vi "DP I-O (Bias).vi"(11 "Expt State (in)":T6) -> (3 "State":T6)   [LabVIEW 2020]
uses:
  CFTS Main Panel SubVIs/CFTS-Data Type Enum.ctl
  Utility VIs/Type Defs/Left-Right ring.ctl
  CFTS Main Panel SubVIs/CFTS-Experiment State.ctl
  Typedefs/DP-StimGen.ctl
  Typedefs/DP-Rejection Settings.ctl
  Typedefs/DP-Stim Params (F1L1).ctl
panel:
  in  "Tab Control":enum32{"Probe tones", "Bias tone"}(tab)
  in  "DP Params":T1={"Start (dB)"=20.0, "Stop (dB)"=70.0, "Step (dB)"=10.0, "Ear"=enum."Right", "f2 (kHz)"="5.6;8.0;11.3;16;22.6;32;", "f1"=1.2, "f1 mode"=enum."re f2", "L1"=10.0, "L1 mode"=enum."re L2"}
  in  "Reject":T3 caption="Rejection"
  in  "StimGen":T4={"Sampling Rate (Hz)"=200000.0, "Npts"=10000, "Data Folder"=path "", "Acoustic System"="", "Recalibrate?"=FALSE, "AO Channels"=[], "Mic  gain (dB)"=0.0, "F1, F2 speakers"=[], "Override recal check"=FALSE}
  out "Freqs":cluster{"f1":dbl, "f2":dbl, "2f1-f2":dbl}={"f1"=9419.759114583332, "f2"=11291.50390625, "2f1-f2"=7548.014322916664} {"2f1-f2" format="%.3f"; "f1" format="%.3f"; "f2" format="%.3f"}
  out "Abort":bool
  in  "Recalibrate":bool
  in  "Probe Mic Gain (dB)":dbl
  in  "Save Waves?":bool=TRUE
  out "User":string
  out "Run #":u16=14
  out "ID #":u16=1
  in  "Avg specs":T5={"# Time avgs "=8, "# Spectrum avgs"=4}
  out "running":bool
  out "Path":path
  out "DP window":cluster{i32, "df (Hz)":dbl, dbl[]}(graph)={0, "df (Hz)"=0.02, []}
  out "I-O Plot":cluster{cluster{dbl, dbl}[]}[](graph)
  in  "Notes":string
  out "Full Spectrum":cluster{i32, "Freq Resolution":dbl, dbl[]}(graph)={0, "Freq Resolution"=20.345052083333332, []}
  in  "RETURN":bool
  in  "START":bool
  in  "STOP":bool
  # "Averaging"
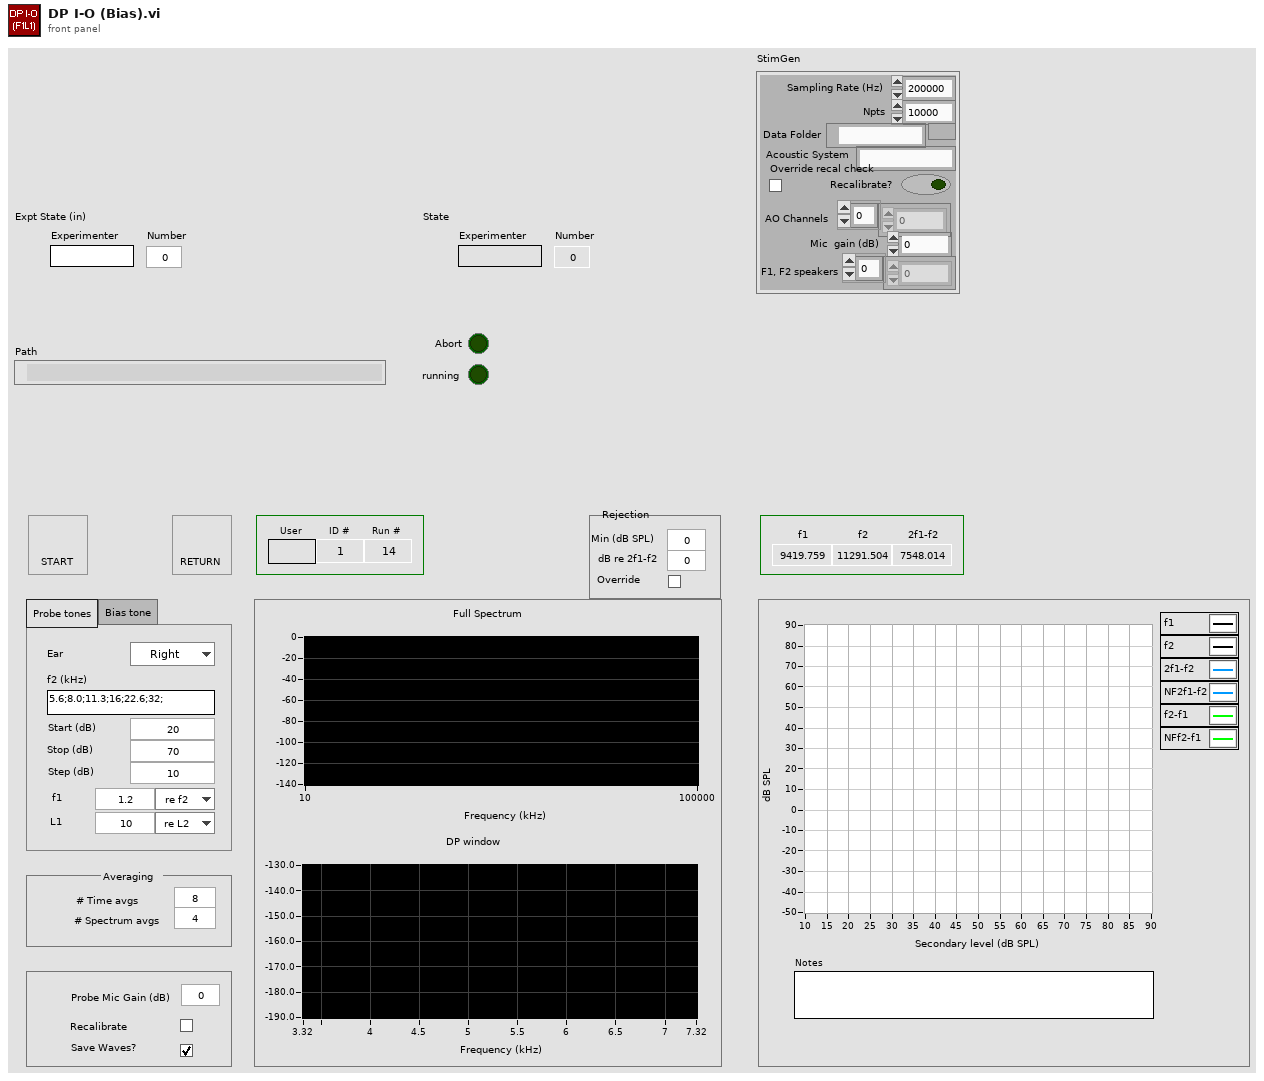
[diagram p1: front panel]
types:
  T1 = typedef "DP-Stim Params (F1L1).ctl" = cluster{"Start (dB)":dbl, "Stop (dB)":dbl, "Step (dB)":dbl, "Ear":T2, "f2 (kHz)":string, "f1":dbl, "f1 mode":enum16{"re f2", "kHz"}, "L1":dbl, "L1 mode":enum16{"re L2", "dB"}}
  T2 = typedef "Left-Right ring.ctl" = enum16{"Right", "Left"}
  T3 = typedef "DP-Rejection Settings.ctl" = cluster{"Override":bool, "dB re 2f1-f2":dbl, "Min (dB SPL)":dbl}
  T4 = typedef "DP-StimGen.ctl" = cluster{"Sampling Rate (Hz)":dbl, "Npts":i32, "Data Folder":path, "Acoustic System":string, "Recalibrate?":bool, "AO Channels":i32[], "Mic  gain (dB)":dbl, "F1, F2 speakers":i32[], "Override recal check":bool}
  T5 = cluster{"# Time avgs ":i32, "# Spectrum avgs":i32}
  T6 = typedef "CFTS-Experiment State.ctl" = cluster{"Experimenter":string, "Number":u32, "Right":string, "Left":string, "Data Folder":path, "State File":path, "Version Info":string, "End Exposure Time":dbl, "Exposure Duration":string, "Run #":cluster{"CAP":i16, "ABR":i16, "DP":i16, "VsEP":i16, "MeasSeq":i16, "SubSeq":i16, "SFOAE":i16}}
  T7 = typedef "CFTS-Data Type Enum.ctl" = enum16{"CAP", "ABR", "DP", "VsEP", "MeasSeq", "SFOAE"}
  T8 = typedef "DP-Freqs.ctl" = cluster{"f1":dbl, "f2":dbl, "2f1-f2":dbl}
  T9 = typedef "DP-DataAcq.ctl" = cluster{"#spectra avgs":i32[], "#time avgs":i32[], "dt (ms)":dbl, "df (kHz)":dbl, "Npts":i32, "Save waves?":bool, "Data File":path, "AI Channels":u16[], "Sampling rate (Hz)":dbl, "Probe Tube Sensitivity":cluster{"Frequency":dbl[], "Mag":dbl[]}, "Mic gain (dB)":dbl, "ptIndex":i32}
  T10 = typedef "CFTS-Options.ctl" = cluster{"DP Artifact Rejection":bool, "Monitor vital signs ":bool, "Extension":string}
  T11 = cluster{"Shift":bool, "Ctrl":bool, "Alt":bool, "Cmd":bool, "Opt":bool}
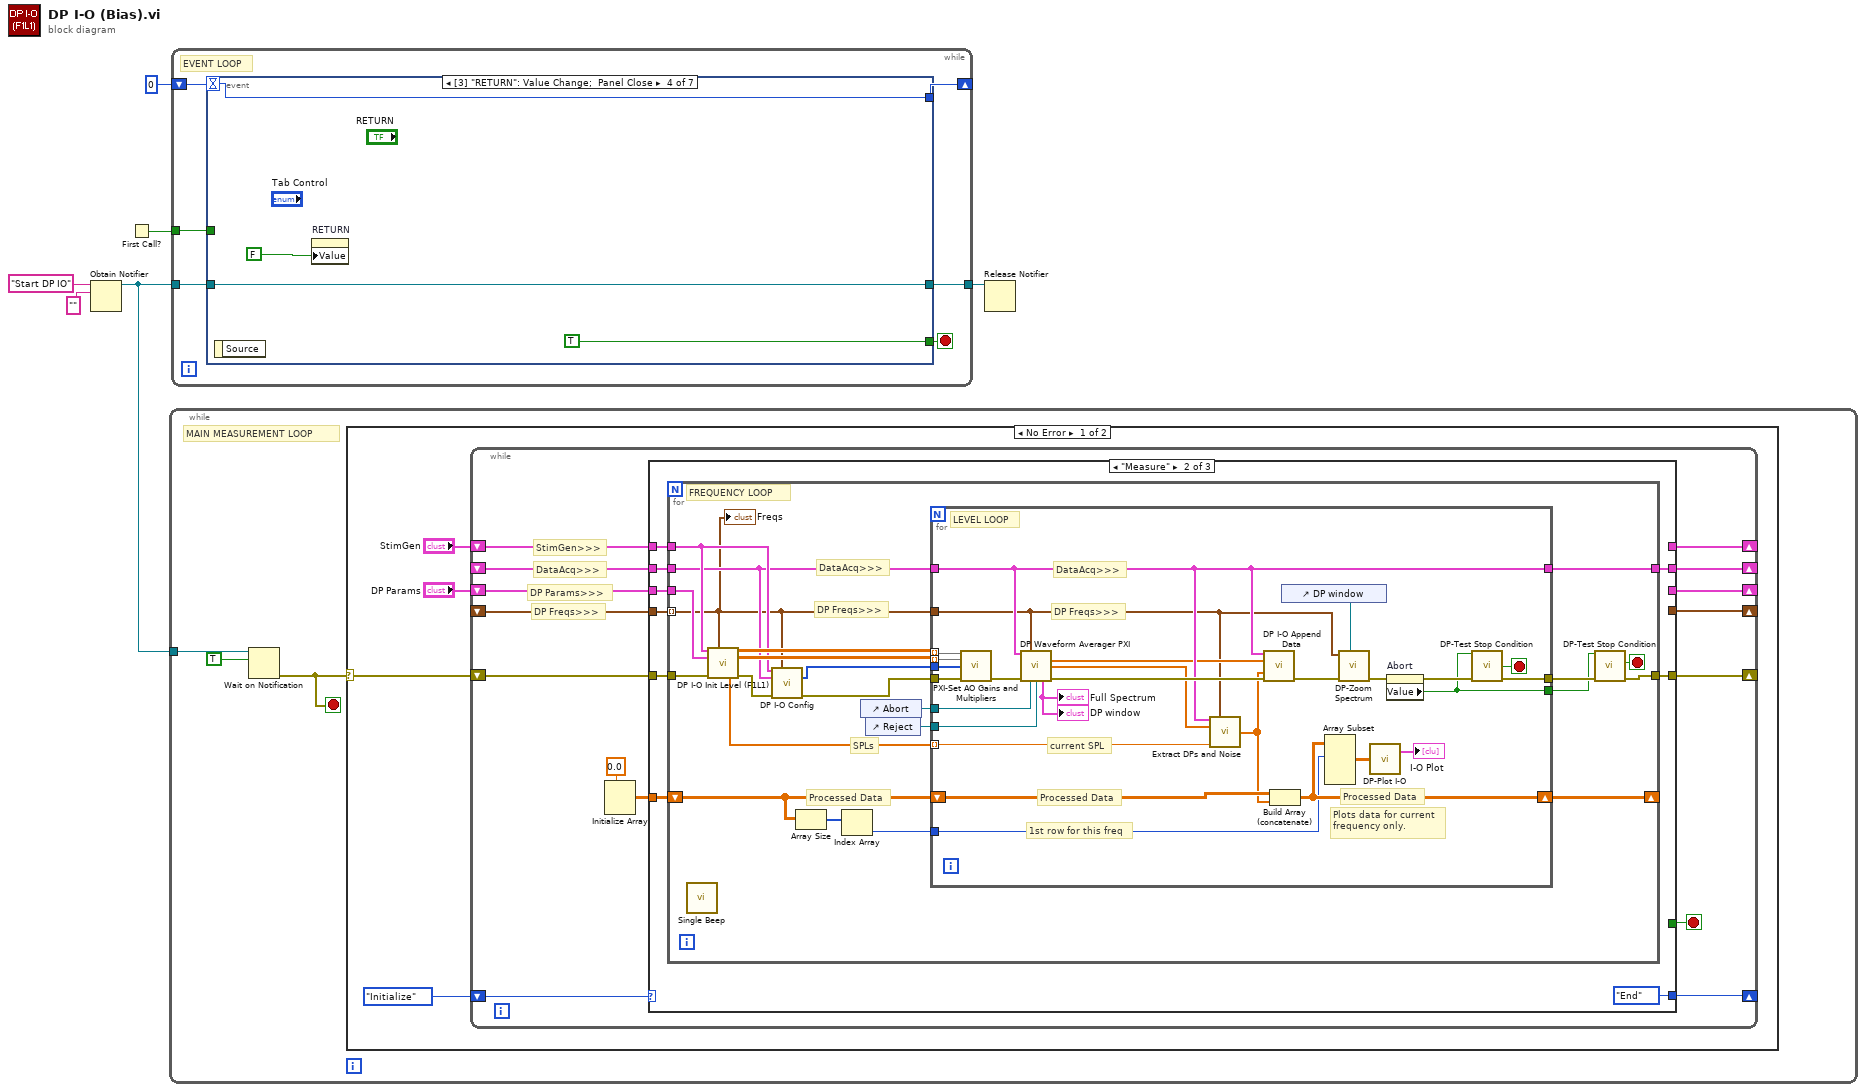
[diagram p0: block diagram]
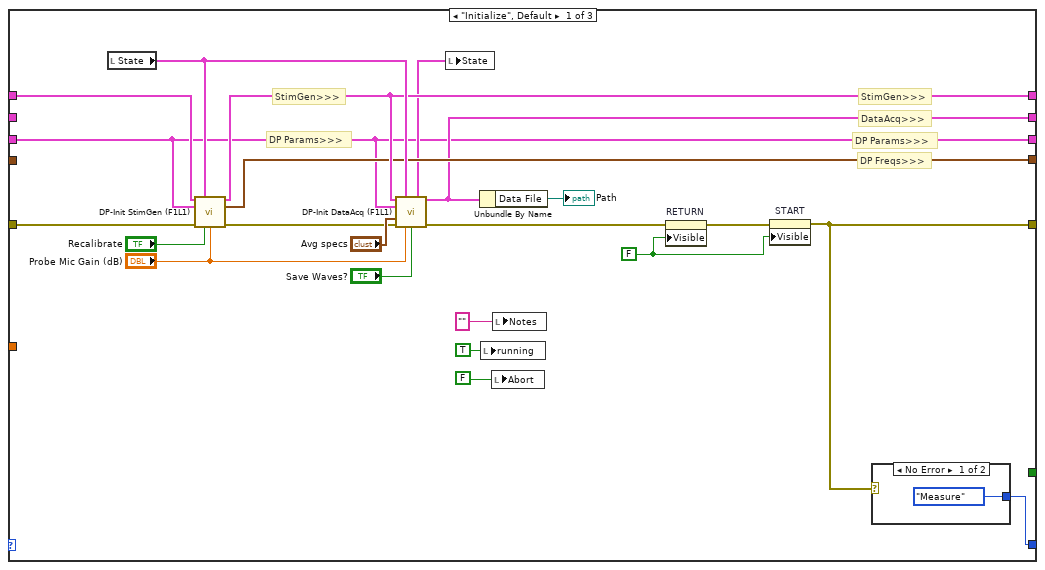
[diagram p2: hidden frame]
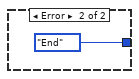
[diagram p3: hidden frame]
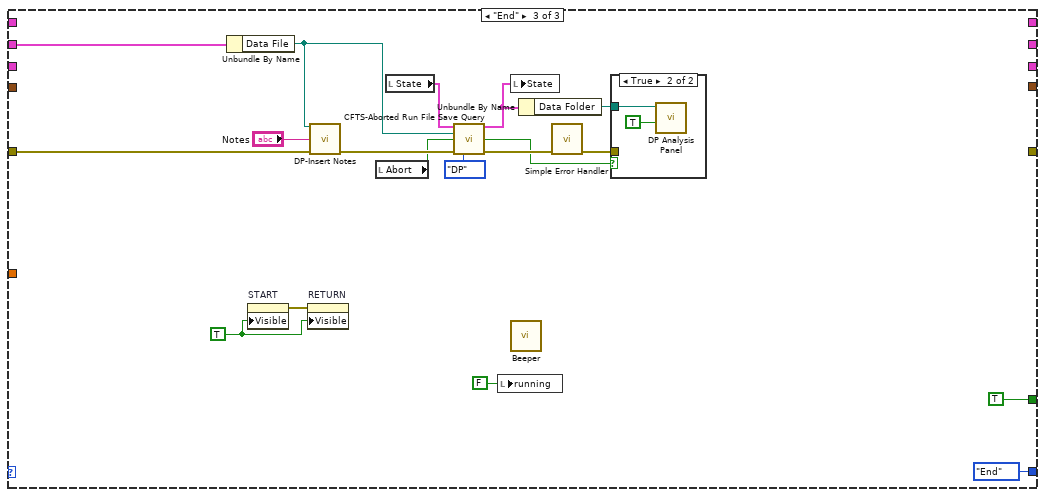
[diagram p4: hidden frame]
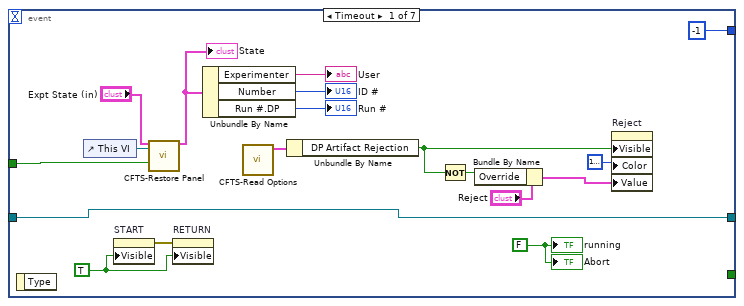
[diagram p7: hidden frame]
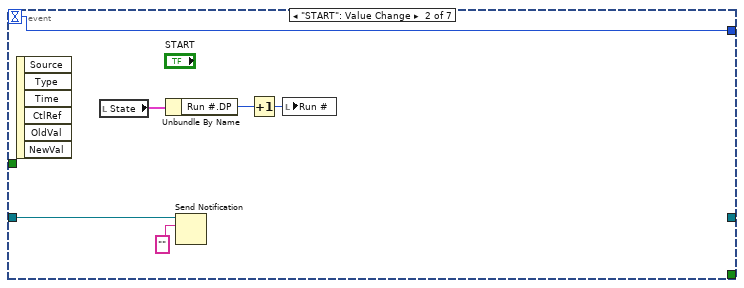
[diagram p8: hidden frame]
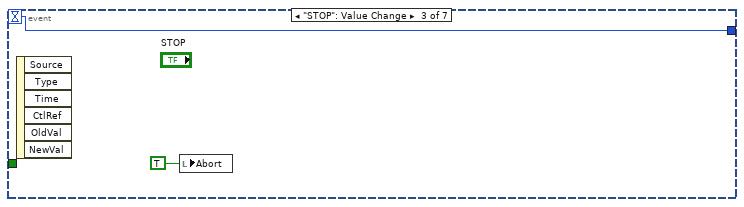
[diagram p9: hidden frame]
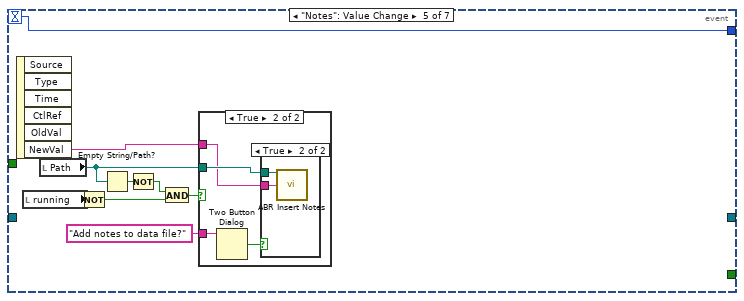
[diagram p10: hidden frame]
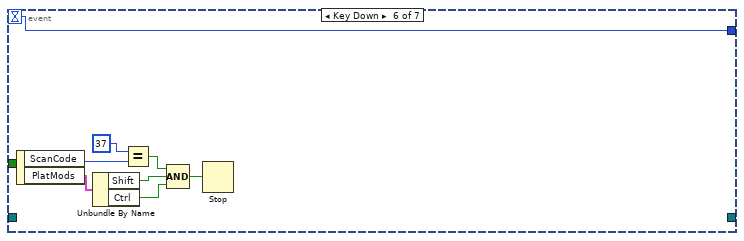
[diagram p13: hidden frame]
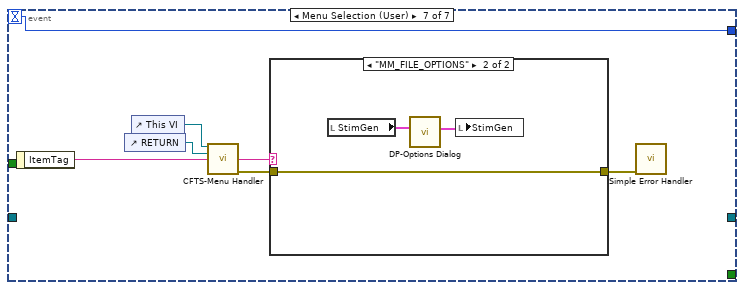
[diagram p14: hidden frame]
diagram:
  n1 = Obtain Notifier(name (unnamed)="Start DP IO", notification data type="") -> (notifier out=w6:refnum<notifier>)  [unwired: 2 in, 2 out]
  n2 = First Call?() -> (First Call?: T/F=w1:bool)
  n3 = while {
    tunnel: w6 -> [w8]
    stop <- w7 stop-if-true
    # "MAIN MEASUREMENT LOOP"
    n4 = Wait on Notification(notifier=w8, ignore previous (F)=TRUE) -> (error out=w7:errorcluster)  [unwired: 2 in, 3 out]
    n5 = case shown="No Error" w7 {
      selector: w7 -> [w10 _]
      frame No Error {
        n6 = while {
          shift-right: [w27] -> _
          shift-left: w10 -> [w28]
          shift-right: [w18] -> _
          shift-left: enum16{"Initialize", "Measure", "End"}."Initialize" -> [w26]
          shift-right: [w22] -> _
          shift-left: "StimGen" -> [w24]
          shift-right: [w21] -> _
          shift-left: _ -> [w23]
          shift-right: [w19] -> _
          shift-left: "DP Params" -> [w20]
          shift-right: [w17] -> _
          shift-left: _ -> [w16]
          stop <- w25 stop-if-true
          # "DP Freqs>>>"
          # "DP Params>>>"
          # "DataAcq>>>"
          # "StimGen>>>"
          n7 = Initialize Array(0.0) -> (w14:dbl[][])  [unwired: 2 in]
          n8 = case shown="\"Measure\"" w26 {
            tunnel: w28 -> [w41 w61 w120]
            tunnel: [w31 w60 _] -> w27
            tunnel: [_ _ TRUE] -> w25
            tunnel: w24 -> [w43 w57 _]
            tunnel: w23 -> [_ w55 w121]
            tunnel: [w42 _ _] -> w22
            tunnel: [w33 w53 _] -> w21
            tunnel: w20 -> [w29 w56 _]
            tunnel: [w29 _ _] -> w19
            tunnel: [w30 enum16{"Initialize", "Measure", "End"}."End" enum16{"Initialize", "Measure", "End"}."End"] -> w18
            tunnel: [w36 _ _] -> w17
            tunnel: w16 -> [_ w58 _]
            tunnel: w14 -> [_ w59 _]
            frame "Initialize", Default {
              w47 = FALSE
              # "DP Freqs>>>"
              # "DP Params>>>"
              # "StimGen>>>"
              # "DP Params>>>"
              # "DataAcq>>>"
              # "StimGen>>>"
              n9 = local read "State"() -> (w44:T6)
              n10 = call "DP-Init StimGen (F1L1).vi"("StimGen"=w43, "Expt State"=w44, "DP stimulus params"=w29, "error in (no error)"=w41, "Recalibrate?"="Recalibrate", "Mic  gain (dB)"="Probe Mic Gain (dB)") -> ("StimGen (out)"=w42:T4, "DP Freqs"=w36:T8[], "error out"=w40:errorcluster)  [unwired: 7 in]
              n11 = call "DP-Init DataAcq (F1L1).vi"("StimGen"=w42, "Expt State"=w44, "DP stimulus params"=w29, "Avg specs"="Avg specs", "error in (no error)"=w40, "Mic gain (dB)"="Probe Mic Gain (dB)", "Save waves?"="Save Waves?") -> ("Expt State out"=w34:T6, "DataAcq"=w33:T9, "error out"=w38:errorcluster)  [unwired: 6 in]
              n12 = local write "State"(w34) -> ()
              n13 = Unbundle By Name(w33) -> ("Data File"=→"Path":path)
              n14 = local write "running"(TRUE ("running")) -> ()
              n15 = local write "Abort"(FALSE ("Stopping")) -> ()
              n16 = local write "Notes"("" ("Notes")) -> ()
              n17 = property on="RETURN" class="Bool (strict)"(error in=w38, "Visible"=w47) -> (error out=w37:errorcluster)  [unwired: 1 in, 1 out]
              n18 = property on="START" class="Bool"(error in=w37, "Visible"=w47) -> (error out=w31:errorcluster)  [unwired: 1 in, 1 out]
              n19 = case shown="No Error" w31 {
                tunnel: [enum16{"Initialize", "Measure", "End"}."Measure" enum16{"Initialize", "Measure", "End"}."End"] -> w30
                frame No Error {
                }
                frame Error {
                }
              }
            }
            frame "Measure" {
              n20 = for {
                shift-right: [w74] -> _
                shift-left: w59 -> [w81]
                tunnel: w61 -> [w78]
                tunnel: [w65] -> w60
                tunnel: w58 -> [w69] mode=indexing
                tunnel: w57 -> [w71]
                tunnel: w56 -> [w73]
                tunnel: w55 -> [w70]
                tunnel: [w68] -> w53
                stop <- w72 stop-if-true
                # "DP Freqs>>>"
                # "DataAcq>>>"
                # "FREQUENCY LOOP"
                # "Processed Data"
                # "SPLs"
                n21 = call "Single Beep.vi"() -> ()  [unwired: 1 in]
                n22 = call "DP I-O Init Level (F1L1).vi"("StimGen"=w71, "DP Freqs"=w69, "DP stimulus params"=w73, "error in (no error)"=w78) -> ("Multipliers (2D)"=w83:dbl[][], "Gains (2D)"=w82:dbl[][], "Nominal f2 SPL"=w75:dbl[], "error out"=w77:errorcluster)  [unwired: 7 in, 1 out]
                n23 = call "DP I-O Config.vi"("StimGen"=w71, "DP Freqs"=w69, "DataAcq"=w70, "error in (no error)"=w77) -> ("AO Channels"=w67:i32[], "error out"=w76:errorcluster)  [unwired: 10 in]
                n24 = Array Size(array=w81) -> (size(s)=w80:i32[])
                n25 = Index Array(array=w80) -> (element=w79:i32)  [unwired: 1 in]
                n26 = control-ref of="Abort"() -> (w63:refnum<vi>)
                n27 = control-ref of="Reject"() -> (w62:refnum<vi>)
                n28 = for {
                  tunnel: w83 -> [w109] mode=indexing
                  tunnel: w82 -> [w108] mode=indexing
                  tunnel: w75 -> [w95] mode=indexing
                  shift-right: [w105] -> w74
                  shift-left: w81 -> [w107]
                  tunnel: w79 -> [w103]
                  tunnel: w76 -> [w110]
                  tunnel: [w90] -> w66
                  tunnel: w70 -> [w94]
                  tunnel: w69 -> [w86]
                  tunnel: [w94] -> w68
                  tunnel: w67 -> [w91]
                  tunnel: [w87] -> w64
                  tunnel: w63 -> [w85]
                  tunnel: w62 -> [w84]
                  stop <- w101 stop-if-true
                  # "DP Freqs>>>"
                  # "DataAcq>>>"
                  # "LEVEL LOOP"
                  # "current SPL"
                  # "Plots data for current\nfrequency only."
                  # "1st row for this freq"
                  # "Processed Data"
                  # "Processed Data"
                  n29 = call "PXI-Set AO Gains and Multipliers.vi"("Multipliers"=w109, "Gains"=w108, "AO Channels"=w91, "error in (no error)"=w110) -> ("error out"=w100:errorcluster)  [unwired: 11 in]
                  n30 = call "DP Waveform Averager PXI.vi"("DataAcq"=w94, "DP Freqs"=w86, "error in"=w100, "Abort"=w85, "Reject Ref"=w84) -> ("Ave Wave"=w93:dbl[], "Averaged Spectrum (Vrms)"=w97:dbl[], "waveform cluster"=→"Full Spectrum" →"DP window":cluster{i32, "dx":dbl, "Array":dbl[]}, "error out"=w99:errorcluster)  [unwired: 5 in, 2 out]
                  n31 = call "Extract DPs and Noise.vi"("DataAcq"=w94, "DP Freqs"=w86, "Spectrum in Vrms"=w97, "SPL"=w95) -> ("Output Array"=w96:dbl[])  [unwired: 11 in]
                  n32 = call "DP I-O Append Data.vi"("DataAcq"=w94, "Waveform"=w93, "Processed data"=w96, "error in (no error)"=w99) -> ("error out"=w102:errorcluster)  [unwired: 11 in]
                  n33 = Build Array (concatenate)(w107, w96) -> (w105:dbl[][])
                  n34 = control-ref of="DP window"() -> (w92:refnum<vi>)
                  n35 = Array Subset(array=w105, index (row)=w103) -> (w104:dbl[][])  [unwired: 3 in]
                  n36 = call "DP-Zoom Spectrum.vi"("DP window"=w92, "error in (no error)"=w102, "DP Freqs"=w86) -> ("error out"=w89:errorcluster)  [unwired: 8 in]
                  n37 = call "DP-Plot I-O.vi"("Input Array (4xn)"=w104) -> ("Current I-O Plot"=→"I-O Plot":cluster{cluster{dbl, dbl}[]}[])  [unwired: 1 out]
                  n38 = property on="Abort" class="Bool (strict)"(error in=w89) -> (error out=w88:errorcluster, "Value"=w87:bool)  [unwired: 1 in, 1 out]
                  n39 = call "DP-Test Stop Condition.vi"("Abort?"=w87, "error in (no error)"=w88) -> ("Stop?"=w101:bool, "error out"=w90:errorcluster)  [unwired: 12 in]
                }
                n40 = call "DP-Test Stop Condition.vi"("Abort?"=w64, "error in (no error)"=w66) -> ("Stop?"=w72:bool, "error out"=w65:errorcluster)  [unwired: 12 in]
                "Freqs" <- w69
              }
            }
            frame "End" {
              w127 = TRUE
              n41 = Unbundle By Name(w121) -> ("Data File"=w117:path)
              n42 = property on="START" class="Bool"("Visible"=w127) -> (error out=w123:errorcluster)  [unwired: 2 in, 1 out]
              n43 = property on="RETURN" class="Bool (strict)"(error in=w123, "Visible"=w127) -> ()  [unwired: 1 in, 2 out]
              n44 = call "DP-Insert Notes.vi"("path"=w117, "Notes"="Notes", "error in (no error)"=w120) -> ("error out"=w122:errorcluster)  [unwired: 12 in]
              n45 = local read "Abort"() -> (w115:bool)
              n46 = local read "State"() -> (w118:T6)
              n47 = call "CFTS-Aborted Run File Save Query.vi"("Expt State"=w118, "Path"=w117, "Aborted"=w115, "error in (no error)"=w122, "Data Type"=CFTS-Data_Type_Enum."DP") -> ("Expt State out"=w114:T6, "File saved?"=w112:bool, "error out"=w119:errorcluster)  [unwired: 8 in]
              n48 = local write "running"(FALSE ("running")) -> ()
              n49 = local write "State"(w114) -> ()
              n50 = call "Beeper.vi"() -> ()  [unwired: 1 in]
              n51 = Unbundle By Name(w114) -> ("Data Folder"=w113:path)
              n52 = call <vilib>:"Simple Error Handler.vi"("error in (no error)"=w119) -> ("error out"=w111:errorcluster)  [unwired: 4 in, 4 out]
              n53 = case shown="True" w112 {
                tunnel: w113 -> [_ w130]
                tunnel: w111 -> [_ _]
                frame False {
                }
                frame True {
                  n54 = call "DP Analysis Panel.vi"("Autosave? (F)"=TRUE, "Data folder in"=w130) -> ()  [unwired: 10 in]
                }
              }
            }
          }
        }
      }
      frame Error {
      }
    }
  }
  n55 = while {
    tunnel: w6 -> [w136]
    shift-right: [w133] -> _
    shift-left: 0 -> [w134]
    tunnel: [w132] -> w2
    tunnel: w1 -> [w131]
    stop <- w135 stop-if-true
    # "EVENT LOOP"
    n56 = event shown="[3] \"RETURN\": Value Change;  Panel Close" {
      selector: _ -> [_ _ _ _ _ _ _]
      dyn-events: _ -> [_ _ _ _ _ _ _]
      timeout: w134 -> [_ w155 w162 w165 w167 w189 w196]
      tunnel: w136 -> [w147 w160 _ w164 _ _ _]
      tunnel: [_ _ _ TRUE _ _ _] -> w135
      tunnel: [-1 w155 w162 w165 w167 w189 w196] -> w133
      tunnel: [w147 _ _ w164 _ _ _] -> w132
      tunnel: w131 -> [w146 _ _ _ _ _ _]
      event Timeout {
        w150 = TRUE
        w149 = FALSE ("quitting")
        n57 = event-data() -> ()  [unwired: 1 in, 1 out]
        n58 = control-ref of="This VI"() -> (w145:refnum<vi>)
        n59 = property on="START" class="Bool"("Visible"=w150) -> (error out=w148:errorcluster)  [unwired: 2 in, 1 out]
        n60 = call "CFTS-Restore Panel.vi"("State (in)"="Expt State (in)", "VI refnum"=w145, "Restore?"=w146) -> ("State"=w143:T6)  [unwired: 11 in, 1 out]
        "State" <- w143
        n61 = property on="RETURN" class="Bool (strict)"(error in=w148, "Visible"=w150) -> ()  [unwired: 1 in, 2 out]
        n62 = Unbundle By Name(w143) -> ("Experimenter"=→"User":string, "Number"=→"ID #":u32, "Run #.DP"=→"Run #":i16)
        n63 = call "CFTS-Read Options.vi"() -> ("CFTS Options"=w142:T10)  [unwired: 10 in, 1 out]
        n64 = Unbundle By Name(w142) -> ("DP Artifact Rejection"=w138:bool)
        n65 = Not(x=w138) -> (.not. x?=w139:bool)
        n66 = Bundle By Name(cluster="Reject", "Override"=w139) -> (w137:T3)
        n67 = property on="Reject" class="Clust (strict)"("Visible"=w138, "Color"=u32 16777238, "Value"=w137) -> ()  [unwired: 2 in, 2 out]
        "running" <- w149
        "Abort" <- w149
      }
      event "START": Value Change {
        n68 = event-data() -> ()  [unwired: 1 in, 6 out]
        n69 = local read "State"() -> (w157:T6)
        n70 = Unbundle By Name(w157) -> ("Run #.DP"=w156:i16)
        n71 = Send Notification(notification="", notifier=w160) -> ()  [unwired: 1 in, 2 out]
        n72 = Increment(x=w156) -> (x+1=w158:i16)
        n73 = local write "Run #"(w158) -> ()
      }
      event "STOP": Value Change {
        n74 = event-data() -> ()  [unwired: 1 in, 6 out]
        n75 = local write "Abort"(TRUE ("Stopping")) -> ()
      }
      event "RETURN": Value Change; Panel Close {
        n76 = event-data() -> ()  [unwired: 1 in, 1 out]
        n77 = property on="RETURN" class="Bool (strict)"("Value"=FALSE) -> ()  [unwired: 2 in, 2 out]
      }
      event "Notes": Value Change {
        n78 = event-data() -> ("NewVal"=w170:string)  [unwired: 1 in, 5 out]
        n79 = local read "running"() -> (w168:bool)
        n80 = local read "Path"() -> (w169:path)
        n81 = Not(x=w168) -> (.not. x?=w172:bool)
        n82 = Empty String/Path?(string/path=w169) -> (empty?=w171:bool)
        n83 = Not(x=w171) -> (.not. x?=w173:bool)
        n84 = And(x=w173, y=w172) -> (x .and. y?=w174:bool)
        n85 = case shown="True" w174 {
          tunnel: w169 -> [_ w179]
          tunnel: w170 -> [_ w178]
          tunnel: "Add notes to data file?" ("message") -> [_ w177]
          frame False {
          }
          frame True {
            n86 = Two Button Dialog(message=w177) -> (T button?=w176:bool)  [unwired: 2 in]
            n87 = case shown="True" w176 {
              tunnel: w179 -> [_ w181]
              tunnel: w178 -> [_ w180]
              frame False {
              }
              frame True {
                n88 = call "ABR Insert Notes.vi"("path"=w181, "Notes"=w180) -> ()  [unwired: 12 in, 2 out]
              }
            }
          }
        }
      }
      event Key Down {
        n89 = event-data() -> ("ScanCode"=w188:i16, "PlatMods"=w186:T11)  [unwired: 1 in]
        n90 = Unbundle By Name(w186) -> ("Shift"=w184:bool, "Ctrl"=w183:bool)
        n91 = Equal?(x=i16 37 ("y"), y=w188) -> (x = y?=w185:bool)
        n92 = Compound Arithmetic op=AND(w185, w184, w183) -> (w182:bool)
        n93 = Stop(stop? (T)=w182) -> ()
      }
      event Menu Selection (User) {
        n94 = event-data() -> ("ItemTag"=w193:string)  [unwired: 1 in]
        n95 = control-ref of="RETURN"() -> (w195:refnum<vi>)
        n96 = control-ref of="This VI"() -> (w194:refnum<vi>)
        n97 = call "CFTS-Menu Handler.vi"("VI Refnum"=w194, "Return Refnum"=w195, "ItemTag"=w193) -> ("ItemTag out"=w192:string, "error out"=w191:errorcluster)  [unwired: 11 in]
        n98 = case shown="\"MM_FILE_OPTIONS\"" w192 {
          tunnel: w191 -> [w197 w200]
          tunnel: [w197 w200] -> w190
          frame "False", Default {
          }
          frame "MM_FILE_OPTIONS" {
            n99 = local read "StimGen"() -> (w199:T4)
            n100 = call "DP-Options Dialog.vi"("StimGen"=w199) -> ("StimGen out"=w198:T4)  [unwired: 8 in, 2 out]
            n101 = local write "StimGen"(w198) -> ()
          }
        }
        n102 = call <vilib>:"Simple Error Handler.vi"("error in (no error)"=w190) -> ()  [unwired: 4 in, 5 out]
      }
    }
  }
  n103 = Release Notifier(notifier=w2) -> ()  [unwired: 2 in, 3 out]
